vi "7SegmentMod2.vi"() -> ()   [LabVIEW 2014]
doc: "\"Discrete LED demo.vi\" -- Demonstrate a discrete LED connected to a digital output.\n\nInstructions:\n\n-- Click the 'enable blinker' button to toggle between blinking mode\nand static mode.\n-- In static mode, click the 'digital level' button to set the state of the\ndigital output.\n-- The 'digital output state' LED indicator shows the state of the\ndigital output (on = high, off = low)."
uses:
  <vilib>/myRIO/Common/Instrument Driver Framework/myRIO v1.0/UART/vis/myRIO v1.0 Close UART.vi
  <vilib>/Utility/error.llb/Error Cluster From Error Code.vi
  <vilib>/myRIO/Common/Instrument Driver Framework/myRIO v1.0/DIO/vis/myRIO v1.0 Write DIO.vi
  <vilib>/myRIO/Common/Instrument Driver Framework/Utilities/vis/FPGA Ref Manager.vi
  <vilib>/myRIO/Common/Instrument Driver Framework/myRIO v1.0/myRIO v1.0 Reset FPGA.vi
  <vilib>/myRIO/Common/Instrument Driver Framework/myRIO v1.0/IRQ/vis/myRIO v1.0 IRQ Info FGV.vi
  <vilib>/myRIO/Common/Instrument Driver Framework/myRIO v1.0/IRQ/vis/myRIO v1.0 Timer IRQ Info FGV.vi
  <vilib>/myRIO/Common/Instrument Driver Framework/myRIO v1.0/IRQ/vis/myRIO v1.0 ISR Agent.vi
  <vilib>/myRIO/Instrument Drivers/Utilities/Utilities.lvlib
  <vilib>/myRIO/Instrument Drivers/Onboard IO/DIO/DIO.lvlib
panel:
  in  "Numeric":u32
  in  "Channel":tag[](array[tag])=["B/DIO0", "B/DIO1", "B/DIO2", "B/DIO3", "B/DIO4", "B/DIO5", "B/DIO6", "B/DIO7"]
  out "error out":errorcluster
  in  "error in (no error)":errorcluster
  in  "[ESC]":bool
  # "7-Segment LED demo"
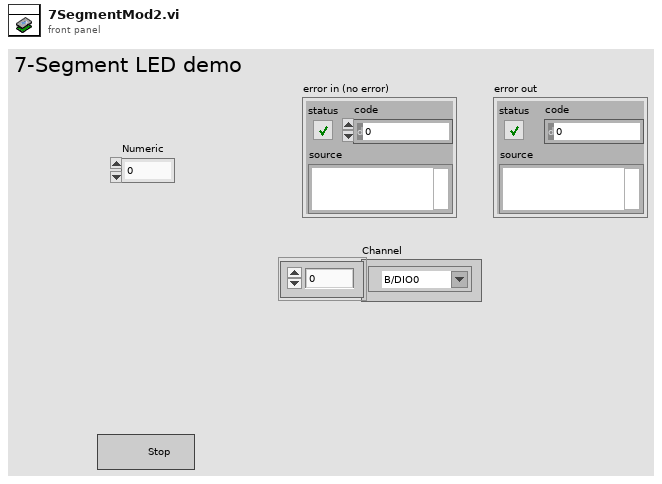
[diagram p1: front panel]
types:
  T1 = typedef "DIO.lvlib/DIO Reference.ctl" = cluster{"myRIO Reference":T2, "DIO Channels List":T6}
  T2 = typedef "myRIO Generic Hardware Reference.ctl" = cluster{"myRIO Model":T3, "myRIO Hardware Reference":T4}
  T3 = typedef "Hardware Version Enum.ctl" = enum16{"Unknown", "myRIO-1900", "myRIO-1950"}
  T4 = typedef "myRIO v1.0 Reference.ctl" = cluster{"Generic FPGA Reference":T5, "Allow multiple opens":bool}
  T5 = typedef "Generic FPGA Reference.ctl" = refnum<k20>
  T6 = typedef "DIO Channels List.ctl" = T7[]
  T7 = typedef "DIO Channels Enum.ctl" = enum16{"Not Connected", "C/DIO0", "C/DIO1", "C/DIO2", "C/DIO3", "C/DIO4", "C/DIO5", "C/DIO6", "C/DIO7", "A/DIO0", "A/DIO1", "A/DIO2", "A/DIO3", "A/DIO4", "A/DIO5", "A/DIO6", "A/DIO7", "A/DIO8", "A/DIO9", "A/DIO10", "A/DIO11", "A/DIO12", "A/DIO13", "A/DIO14", "A/DIO15", "B/DIO0", "B/DIO1", "B/DIO2", "B/DIO3", "B/DIO4", "B/DIO5", "B/DIO6", "B/DIO7", "B/DIO8", "B/DIO9", "B/DIO10", "B/DIO11", "B/DIO12", "B/DIO13", "B/DIO14", "B/DIO15", "LED0", "LED1", "LED2", "LED3", "Button0"}
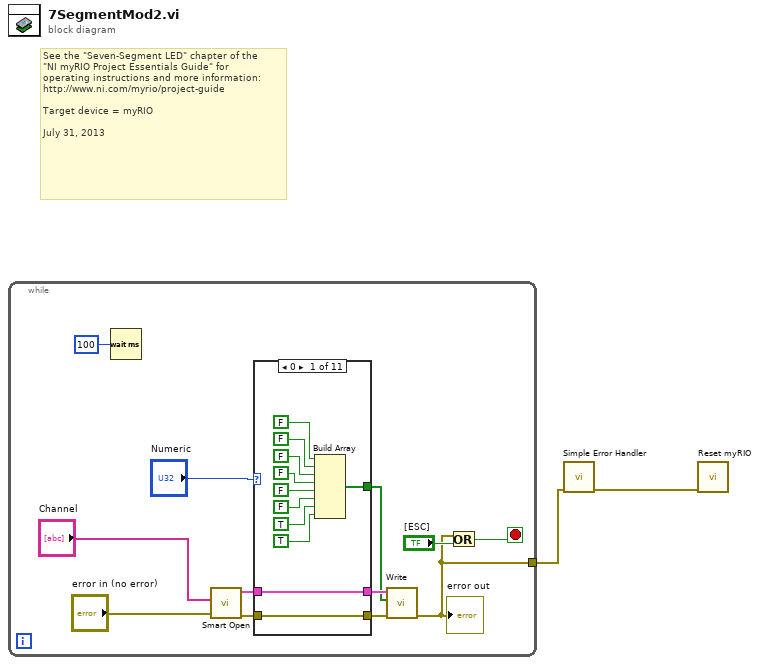
[diagram p0: block diagram]
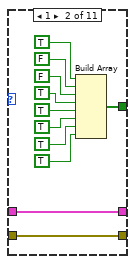
[diagram p2: hidden frame]
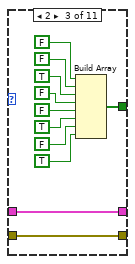
[diagram p3: hidden frame]
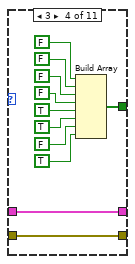
[diagram p4: hidden frame]
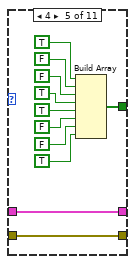
[diagram p5: hidden frame]
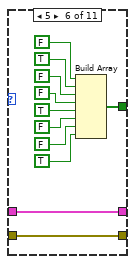
[diagram p6: hidden frame]
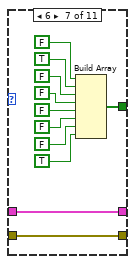
[diagram p7: hidden frame]
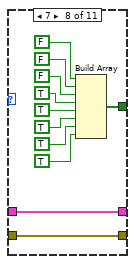
[diagram p8: hidden frame]
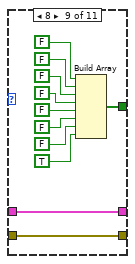
[diagram p9: hidden frame]
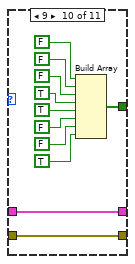
[diagram p10: hidden frame]
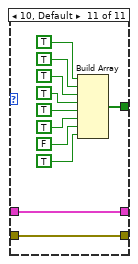
[diagram p11: hidden frame]
diagram:
  # "See the \"Seven-Segment LED\" chapter of the\n\"NI myRIO Project Essentials Guide\" for\noperating instructions and more information: \nhttp://www.ni.com/myrio/project-guide\n\nTarget device = myRIO\n\nJuly 31, 2013"
  n1 = while {
    tunnel: [w9] -> w1
    stop <- w14 stop-if-true
    n2 = Wait (ms)(milliseconds to wait=u32 100) -> ()  [unwired: 1 out]
    n3 = call <vilib>:"Smart Open.vi"("error in (no error)"="error in (no error)", "Channel Names"="Channel") -> ("error out"=w6:errorcluster, "DIO Ref Out"=w8:T1)  [unwired: 8 in]
    n4 = case shown="0" "Numeric" {
      tunnel: w8 -> [w16 w28 w39 w50 w61 w72 w83 w94 w105 w116 w127]
      tunnel: [w16 w28 w39 w50 w61 w72 w83 w94 w105 w116 w127] -> w7
      tunnel: w6 -> [w15 w27 w38 w49 w60 w71 w82 w93 w104 w115 w126]
      tunnel: [w15 w27 w38 w49 w60 w71 w82 w93 w104 w115 w126] -> w5
      tunnel: [w17 w26 w37 w48 w59 w70 w81 w92 w103 w114 w125] -> w3
      frame 0 {
        n5 = Build Array(FALSE, FALSE, FALSE, FALSE, FALSE, FALSE, TRUE, TRUE) -> (w17:bool[])
      }
      frame 1 {
        n6 = Build Array(TRUE, FALSE, FALSE, TRUE, TRUE, TRUE, TRUE, TRUE) -> (w26:bool[])
      }
      frame 2 {
        n7 = Build Array(FALSE, FALSE, TRUE, FALSE, FALSE, TRUE, FALSE, TRUE) -> (w37:bool[])
      }
      frame 3 {
        n8 = Build Array(FALSE, FALSE, FALSE, FALSE, TRUE, TRUE, FALSE, TRUE) -> (w48:bool[])
      }
      frame 4 {
        n9 = Build Array(TRUE, FALSE, FALSE, TRUE, TRUE, FALSE, FALSE, TRUE) -> (w59:bool[])
      }
      frame 5 {
        n10 = Build Array(FALSE, TRUE, FALSE, FALSE, TRUE, FALSE, FALSE, TRUE) -> (w70:bool[])
      }
      frame 6 {
        n11 = Build Array(FALSE, TRUE, FALSE, FALSE, FALSE, FALSE, FALSE, TRUE) -> (w81:bool[])
      }
      frame 7 {
        n12 = Build Array(FALSE, FALSE, FALSE, TRUE, TRUE, TRUE, TRUE, TRUE) -> (w92:bool[])
      }
      frame 8 {
        n13 = Build Array(FALSE, FALSE, FALSE, FALSE, FALSE, FALSE, FALSE, TRUE) -> (w103:bool[])
      }
      frame 9 {
        n14 = Build Array(FALSE, FALSE, FALSE, TRUE, TRUE, FALSE, FALSE, TRUE) -> (w114:bool[])
      }
      frame 10, Default {
        n15 = Build Array(TRUE, TRUE, TRUE, TRUE, TRUE, TRUE, FALSE, TRUE) -> (w125:bool[])
      }
    }
    n16 = call <vilib>:"Write.vi"("error in (no error)"=w5, "Values"=w3, "DIO Ref In"=w7) -> ("error out"=w9:errorcluster)  [unwired: 6 in, 1 out]
    "error out" <- w9
    n17 = Or(x=w9, y="[ESC]") -> (x .or. y?=w14:bool)
  }
  n18 = call <vilib>:"Simple Error Handler.vi"("error in (no error)"=w1) -> ("error out"=w2:errorcluster)  [unwired: 4 in, 4 out]
  n19 = call <vilib>:"Reset myRIO.vi"("error in (no error)"=w2) -> ()  [unwired: 10 in, 1 out]
